vi "Pulses to Radians.vi"(10 "gear ratio":dbl, 11 "encoder pulses":i32) -> (3 "angle (rad)":dbl)   [LabVIEW 2011, in "MF3.lvclass"]
uses:
  MF3.lvclass
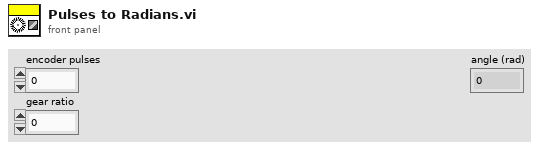
[diagram p1: front panel]
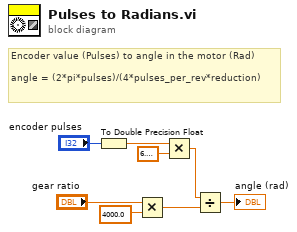
[diagram p0: block diagram]
diagram:
  # "Encoder value (Pulses) to angle in the motor (Rad)\n\nangle = (2*pi*pulses)/(4*pulses_per_rev*reduction)"
  n1 = To Double Precision Float(number="encoder pulses") -> (double precision float=w7:dbl)
  n2 = Multiply(x="gear ratio", y=4000.0 ("x")) -> (x*y=w2:dbl)
  n3 = Multiply(x=w7, y=6.283185307179586) -> (x*y=w5:dbl)
  n4 = Divide(x=w5, y=w2) -> (x/y=→"angle (rad)":dbl)
